vi "VI Gaszuordnung.vi"() -> ()   [LabVIEW 2020, in "Gaszuordnung AO.lvlib"]
uses:
  Seiten/Gaszuordnung AO/Gaszuordnung AO.lvlib
  Seiten/Gaszuordnung AO/Auswahlfelder Anzeige.ctl
  Visualisierungs Elemente/Auswahlfeld.ctl
  Seiten/Gaszuordnung AO/Aktuelle Werte Anzeige.ctl
  Seiten/Gaszuordnung AO/Grenzen Anzeige.ctl
  Visualisierungs Elemente/Zahlen-Eingabefeld.ctl
  Seiten/Gaszuordnung AO/Einheit Anzeige.ctl
  Visualisierungs Elemente/String - Ausgabefeld.ctl
  Seiten/Gaszuordnung AO/Balken Anzeige.ctl
  Seiten/Gaszuordnung AO/Balken.ctl
  Visualisierungs Elemente/Button.ctl
  Seiten/Gaszuordnung AO/FGV Gaszuordnung Gas-Auswahl Aktion.ctl
  Seiten/FT-IR/FGV FT-IR Gasliste Aktionen.ctl
  Passwortverwaltung/FGV Passwort Aktion.ctl
  Seiten/Gaszuordnung AO/FGV Gaszuordnung Grenzen&Einheit Aktion.ctl
  Seiten/FT-IR/FT-IR.lvlib
  Passwortverwaltung/Passwort.lvlib
  Allgemein/allgemeine Sub-VIs.lvlib
panel:
  in  "Grenzw. Speichern":T1
  in  "Grenzen Max":T2 {"Zahlen-Eingabefeld 16" format="%#_5g"; "Zahlen-Eingabefeld 15" format="%#_5g"; "Zahlen-Eingabefeld 14" format="%#_5g"; "Zahlen-Eingabefeld 13" format="%#_5g"; "Zahlen-Eingabefeld 12" format="%#_5g"; "Zahlen-Eingabefeld 11" format="%#_5g"; "Zahlen-Eingabefeld 10" format="%#_5g"; "Zahlen-Eingabefeld 9" format="%#_5g"; "Zahlen-Eingabefeld 8" format="%#_5g"; "Zahlen-Eingabefeld 7" format="%#_5g"; "Zahlen-Eingabefeld 6" format="%#_5g"; "Zahlen-Eingabefeld 5" format="%#_5g"; "Zahlen-Eingabefeld 4" format="%#_5g"; "Zahlen-Eingabefeld 3" format="%#_5g"; "Zahlen-Eingabefeld 2" format="%#_5g"; "Zahlen-Eingabefeld" format="%#_5g"}
  out "Balken Anzeige":T4 {"Anzeige Balken 16" scale=0.0..100.0; "Anzeige Balken 15" scale=0.0..100.0; "Anzeige Balken 14" scale=0.0..100.0; "Anzeige Balken 13" scale=0.0..100.0; "Anzeige Balken 12" scale=0.0..100.0; "Anzeige Balken 11" scale=0.0..100.0; "Anzeige Balken 10" scale=0.0..100.0; "Anzeige Balken 9" scale=0.0..100.0; "Anzeige Balken 8" scale=0.0..100.0; "Anzeige Balken 7" scale=0.0..100.0; "Anzeige Balken 6" scale=0.0..100.0; "Anzeige Balken 5" scale=0.0..100.0; "Anzeige Balken 4" scale=0.0..100.0; "Anzeige Balken 3" scale=0.0..100.0; "Anzeige Balken 2" scale=0.0..100.0; "Anzeige Balken" scale=0.0..100.0}
  out "Einheit Anzeige":T6
  in  "Grenzen Min":T2 {"Zahlen-Eingabefeld 16" format="%#_5g"; "Zahlen-Eingabefeld 15" format="%#_5g"; "Zahlen-Eingabefeld 14" format="%#_5g"; "Zahlen-Eingabefeld 13" format="%#_5g"; "Zahlen-Eingabefeld 12" format="%#_5g"; "Zahlen-Eingabefeld 11" format="%#_5g"; "Zahlen-Eingabefeld 10" format="%#_5g"; "Zahlen-Eingabefeld 9" format="%#_5g"; "Zahlen-Eingabefeld 8" format="%#_5g"; "Zahlen-Eingabefeld 7" format="%#_5g"; "Zahlen-Eingabefeld 6" format="%#_5g"; "Zahlen-Eingabefeld 5" format="%#_5g"; "Zahlen-Eingabefeld 4" format="%#_5g"; "Zahlen-Eingabefeld 3" format="%#_5g"; "Zahlen-Eingabefeld 2" format="%#_5g"; "Zahlen-Eingabefeld" format="%#_5g"}
  out "Aktuelle Werte":T8 {"Zahlen-Ausgabefeld 16" format="%#.2f"; "Zahlen-Ausgabefeld 15" format="%#.2f"; "Zahlen-Ausgabefeld 14" format="%#.2f"; "Zahlen-Ausgabefeld 13" format="%#.2f"; "Zahlen-Ausgabefeld 12" format="%#.2f"; "Zahlen-Ausgabefeld 11" format="%#.2f"; "Zahlen-Ausgabefeld 10" format="%#.2f"; "Zahlen-Ausgabefeld 9" format="%#.2f"; "Zahlen-Ausgabefeld 8" format="%#.2f"; "Zahlen-Ausgabefeld 7" format="%#.2f"; "Zahlen-Ausgabefeld 6" format="%#.2f"; "Zahlen-Ausgabefeld 5" format="%#.2f"; "Zahlen-Ausgabefeld 4" format="%#.2f"; "Zahlen-Ausgabefeld 3" format="%#.2f"; "Zahlen-Ausgabefeld 2" format="%#.2f"; "Zahlen-Ausgabefeld" format="%#.2f"}
  in  "Auswahlfelder":T9 {"Auswahl 16" items=["NO (3000) LP 191C", "NO2 (150) LP 191C (1of2)", "NO2 (2000) LP 191C (2of2)", "N2O (300) LP 191C (1of2)", "NH3 (300) LP 191C (1of2)", "NH3 (900,3000) LP 191C (2of2)", "HNCO (400) 191C", "H2O% (30) LP 191C", "Formaldehyde (70,500) LP 191C", "CO2 low% (4) LP 191C (2of2)", "CO2% (20) LP 191C (1of2)", "CO (700) LP 191C (1of3)", "CO% (1) LP 191C (2of3)", "Propylene (1000) LP 191C", "Aromatic HC C7 (500) LP 191C", "Ethylene (1000) LP 191C", "CH4 (250) LP 191C (1of2)", "CH4 (5000) LP 191C (2of2)", "Ethane (1000) LP 191C", "Acetylene (1000) LP 191C", "HNO2 (20) 191C", "MeOH (1000) 191C", "CO% (10) LP 191C (3of3)", "Formic Acid (100) 191C", "SO2 (500) LP 191C", "Acetaldehyde (1000) LP 191C", "COS (100) LP 191C", "1,3 butadiene (100) LP 191C", "Oil as Octane (200) LP 191C", "N2O (1000) LP 191C (2of2)", "Propane (200) LP 191C", "NO2 autorange (2000)", "CO autorange (100000)", "CH4 autorange (5000)", "NH3 autorange (3000)", "NOx autorange (3000)", "HCD (10000)", "NMHCD (10000)", "CO2% autorange (20)", "H2Oppm (300000)", "N2O autorange (1000)", "NMNEHCD (3000)", "Temp. Gascell", "Pressure Gascell", "sBeam@2500", "Temp. HL to FT-IR", "Temp. HL Extern SP1", "Outlet Temp FT-IR", "Temp. Cabinet", "Constant 0", "Constant 50", "Constant 100", "AK DUMMY"]; "Auswahl 15" items=["NO (3000) LP 191C", "NO2 (150) LP 191C (1of2)", "NO2 (2000) LP 191C (2of2)", "N2O (300) LP 191C (1of2)", "NH3 (300) LP 191C (1of2)", "NH3 (900,3000) LP 191C (2of2)", "HNCO (400) 191C", "H2O% (30) LP 191C", "Formaldehyde (70,500) LP 191C", "CO2 low% (4) LP 191C (2of2)", "CO2% (20) LP 191C (1of2)", "CO (700) LP 191C (1of3)", "CO% (1) LP 191C (2of3)", "Propylene (1000) LP 191C", "Aromatic HC C7 (500) LP 191C", "Ethylene (1000) LP 191C", "CH4 (250) LP 191C (1of2)", "CH4 (5000) LP 191C (2of2)", "Ethane (1000) LP 191C", "Acetylene (1000) LP 191C", "HNO2 (20) 191C", "MeOH (1000) 191C", "CO% (10) LP 191C (3of3)", "Formic Acid (100) 191C", "SO2 (500) LP 191C", "Acetaldehyde (1000) LP 191C", "COS (100) LP 191C", "1,3 butadiene (100) LP 191C", "Oil as Octane (200) LP 191C", "N2O (1000) LP 191C (2of2)", "Propane (200) LP 191C", "NO2 autorange (2000)", "CO autorange (100000)", "CH4 autorange (5000)", "NH3 autorange (3000)", "NOx autorange (3000)", "HCD (10000)", "NMHCD (10000)", "CO2% autorange (20)", "H2Oppm (300000)", "N2O autorange (1000)", "NMNEHCD (3000)", "Temp. Gascell", "Pressure Gascell", "sBeam@2500", "Temp. HL to FT-IR", "Temp. HL Extern SP1", "Outlet Temp FT-IR", "Temp. Cabinet", "Constant 0", "Constant 50", "Constant 100", "AK DUMMY"]; "Auswahl 14" items=["NO (3000) LP 191C", "NO2 (150) LP 191C (1of2)", "NO2 (2000) LP 191C (2of2)", "N2O (300) LP 191C (1of2)", "NH3 (300) LP 191C (1of2)", "NH3 (900,3000) LP 191C (2of2)", "HNCO (400) 191C", "H2O% (30) LP 191C", "Formaldehyde (70,500) LP 191C", "CO2 low% (4) LP 191C (2of2)", "CO2% (20) LP 191C (1of2)", "CO (700) LP 191C (1of3)", "CO% (1) LP 191C (2of3)", "Propylene (1000) LP 191C", "Aromatic HC C7 (500) LP 191C", "Ethylene (1000) LP 191C", "CH4 (250) LP 191C (1of2)", "CH4 (5000) LP 191C (2of2)", "Ethane (1000) LP 191C", "Acetylene (1000) LP 191C", "HNO2 (20) 191C", "MeOH (1000) 191C", "CO% (10) LP 191C (3of3)", "Formic Acid (100) 191C", "SO2 (500) LP 191C", "Acetaldehyde (1000) LP 191C", "COS (100) LP 191C", "1,3 butadiene (100) LP 191C", "Oil as Octane (200) LP 191C", "N2O (1000) LP 191C (2of2)", "Propane (200) LP 191C", "NO2 autorange (2000)", "CO autorange (100000)", "CH4 autorange (5000)", "NH3 autorange (3000)", "NOx autorange (3000)", "HCD (10000)", "NMHCD (10000)", "CO2% autorange (20)", "H2Oppm (300000)", "N2O autorange (1000)", "NMNEHCD (3000)", "Temp. Gascell", "Pressure Gascell", "sBeam@2500", "Temp. HL to FT-IR", "Temp. HL Extern SP1", "Outlet Temp FT-IR", "Temp. Cabinet", "Constant 0", "Constant 50", "Constant 100", "AK DUMMY"]; "Auswahl 13" items=["NO (3000) LP 191C", "NO2 (150) LP 191C (1of2)", "NO2 (2000) LP 191C (2of2)", "N2O (300) LP 191C (1of2)", "NH3 (300) LP 191C (1of2)", "NH3 (900,3000) LP 191C (2of2)", "HNCO (400) 191C", "H2O% (30) LP 191C", "Formaldehyde (70,500) LP 191C", "CO2 low% (4) LP 191C (2of2)", "CO2% (20) LP 191C (1of2)", "CO (700) LP 191C (1of3)", "CO% (1) LP 191C (2of3)", "Propylene (1000) LP 191C", "Aromatic HC C7 (500) LP 191C", "Ethylene (1000) LP 191C", "CH4 (250) LP 191C (1of2)", "CH4 (5000) LP 191C (2of2)", "Ethane (1000) LP 191C", "Acetylene (1000) LP 191C", "HNO2 (20) 191C", "MeOH (1000) 191C", "CO% (10) LP 191C (3of3)", "Formic Acid (100) 191C", "SO2 (500) LP 191C", "Acetaldehyde (1000) LP 191C", "COS (100) LP 191C", "1,3 butadiene (100) LP 191C", "Oil as Octane (200) LP 191C", "N2O (1000) LP 191C (2of2)", "Propane (200) LP 191C", "NO2 autorange (2000)", "CO autorange (100000)", "CH4 autorange (5000)", "NH3 autorange (3000)", "NOx autorange (3000)", "HCD (10000)", "NMHCD (10000)", "CO2% autorange (20)", "H2Oppm (300000)", "N2O autorange (1000)", "NMNEHCD (3000)", "Temp. Gascell", "Pressure Gascell", "sBeam@2500", "Temp. HL to FT-IR", "Temp. HL Extern SP1", "Outlet Temp FT-IR", "Temp. Cabinet", "Constant 0", "Constant 50", "Constant 100", "AK DUMMY"]; "Auswahl 12" items=["NO (3000) LP 191C", "NO2 (150) LP 191C (1of2)", "NO2 (2000) LP 191C (2of2)", "N2O (300) LP 191C (1of2)", "NH3 (300) LP 191C (1of2)", "NH3 (900,3000) LP 191C (2of2)", "HNCO (400) 191C", "H2O% (30) LP 191C", "Formaldehyde (70,500) LP 191C", "CO2 low% (4) LP 191C (2of2)", "CO2% (20) LP 191C (1of2)", "CO (700) LP 191C (1of3)", "CO% (1) LP 191C (2of3)", "Propylene (1000) LP 191C", "Aromatic HC C7 (500) LP 191C", "Ethylene (1000) LP 191C", "CH4 (250) LP 191C (1of2)", "CH4 (5000) LP 191C (2of2)", "Ethane (1000) LP 191C", "Acetylene (1000) LP 191C", "HNO2 (20) 191C", "MeOH (1000) 191C", "CO% (10) LP 191C (3of3)", "Formic Acid (100) 191C", "SO2 (500) LP 191C", "Acetaldehyde (1000) LP 191C", "COS (100) LP 191C", "1,3 butadiene (100) LP 191C", "Oil as Octane (200) LP 191C", "N2O (1000) LP 191C (2of2)", "Propane (200) LP 191C", "NO2 autorange (2000)", "CO autorange (100000)", "CH4 autorange (5000)", "NH3 autorange (3000)", "NOx autorange (3000)", "HCD (10000)", "NMHCD (10000)", "CO2% autorange (20)", "H2Oppm (300000)", "N2O autorange (1000)", "NMNEHCD (3000)", "Temp. Gascell", "Pressure Gascell", "sBeam@2500", "Temp. HL to FT-IR", "Temp. HL Extern SP1", "Outlet Temp FT-IR", "Temp. Cabinet", "Constant 0", "Constant 50", "Constant 100", "AK DUMMY"]; "Auswahl 11" items=["NO (3000) LP 191C", "NO2 (150) LP 191C (1of2)", "NO2 (2000) LP 191C (2of2)", "N2O (300) LP 191C (1of2)", "NH3 (300) LP 191C (1of2)", "NH3 (900,3000) LP 191C (2of2)", "HNCO (400) 191C", "H2O% (30) LP 191C", "Formaldehyde (70,500) LP 191C", "CO2 low% (4) LP 191C (2of2)", "CO2% (20) LP 191C (1of2)", "CO (700) LP 191C (1of3)", "CO% (1) LP 191C (2of3)", "Propylene (1000) LP 191C", "Aromatic HC C7 (500) LP 191C", "Ethylene (1000) LP 191C", "CH4 (250) LP 191C (1of2)", "CH4 (5000) LP 191C (2of2)", "Ethane (1000) LP 191C", "Acetylene (1000) LP 191C", "HNO2 (20) 191C", "MeOH (1000) 191C", "CO% (10) LP 191C (3of3)", "Formic Acid (100) 191C", "SO2 (500) LP 191C", "Acetaldehyde (1000) LP 191C", "COS (100) LP 191C", "1,3 butadiene (100) LP 191C", "Oil as Octane (200) LP 191C", "N2O (1000) LP 191C (2of2)", "Propane (200) LP 191C", "NO2 autorange (2000)", "CO autorange (100000)", "CH4 autorange (5000)", "NH3 autorange (3000)", "NOx autorange (3000)", "HCD (10000)", "NMHCD (10000)", "CO2% autorange (20)", "H2Oppm (300000)", "N2O autorange (1000)", "NMNEHCD (3000)", "Temp. Gascell", "Pressure Gascell", "sBeam@2500", "Temp. HL to FT-IR", "Temp. HL Extern SP1", "Outlet Temp FT-IR", "Temp. Cabinet", "Constant 0", "Constant 50", "Constant 100", "AK DUMMY"]; "Auswahl 10" items=["NO (3000) LP 191C", "NO2 (150) LP 191C (1of2)", "NO2 (2000) LP 191C (2of2)", "N2O (300) LP 191C (1of2)", "NH3 (300) LP 191C (1of2)", "NH3 (900,3000) LP 191C (2of2)", "HNCO (400) 191C", "H2O% (30) LP 191C", "Formaldehyde (70,500) LP 191C", "CO2 low% (4) LP 191C (2of2)", "CO2% (20) LP 191C (1of2)", "CO (700) LP 191C (1of3)", "CO% (1) LP 191C (2of3)", "Propylene (1000) LP 191C", "Aromatic HC C7 (500) LP 191C", "Ethylene (1000) LP 191C", "CH4 (250) LP 191C (1of2)", "CH4 (5000) LP 191C (2of2)", "Ethane (1000) LP 191C", "Acetylene (1000) LP 191C", "HNO2 (20) 191C", "MeOH (1000) 191C", "CO% (10) LP 191C (3of3)", "Formic Acid (100) 191C", "SO2 (500) LP 191C", "Acetaldehyde (1000) LP 191C", "COS (100) LP 191C", "1,3 butadiene (100) LP 191C", "Oil as Octane (200) LP 191C", "N2O (1000) LP 191C (2of2)", "Propane (200) LP 191C", "NO2 autorange (2000)", "CO autorange (100000)", "CH4 autorange (5000)", "NH3 autorange (3000)", "NOx autorange (3000)", "HCD (10000)", "NMHCD (10000)", "CO2% autorange (20)", "H2Oppm (300000)", "N2O autorange (1000)", "NMNEHCD (3000)", "Temp. Gascell", "Pressure Gascell", "sBeam@2500", "Temp. HL to FT-IR", "Temp. HL Extern SP1", "Outlet Temp FT-IR", "Temp. Cabinet", "Constant 0", "Constant 50", "Constant 100", "AK DUMMY"]; "Auswahl 9" items=["NO (3000) LP 191C", "NO2 (150) LP 191C (1of2)", "NO2 (2000) LP 191C (2of2)", "N2O (300) LP 191C (1of2)", "NH3 (300) LP 191C (1of2)", "NH3 (900,3000) LP 191C (2of2)", "HNCO (400) 191C", "H2O% (30) LP 191C", "Formaldehyde (70,500) LP 191C", "CO2 low% (4) LP 191C (2of2)", "CO2% (20) LP 191C (1of2)", "CO (700) LP 191C (1of3)", "CO% (1) LP 191C (2of3)", "Propylene (1000) LP 191C", "Aromatic HC C7 (500) LP 191C", "Ethylene (1000) LP 191C", "CH4 (250) LP 191C (1of2)", "CH4 (5000) LP 191C (2of2)", "Ethane (1000) LP 191C", "Acetylene (1000) LP 191C", "HNO2 (20) 191C", "MeOH (1000) 191C", "CO% (10) LP 191C (3of3)", "Formic Acid (100) 191C", "SO2 (500) LP 191C", "Acetaldehyde (1000) LP 191C", "COS (100) LP 191C", "1,3 butadiene (100) LP 191C", "Oil as Octane (200) LP 191C", "N2O (1000) LP 191C (2of2)", "Propane (200) LP 191C", "NO2 autorange (2000)", "CO autorange (100000)", "CH4 autorange (5000)", "NH3 autorange (3000)", "NOx autorange (3000)", "HCD (10000)", "NMHCD (10000)", "CO2% autorange (20)", "H2Oppm (300000)", "N2O autorange (1000)", "NMNEHCD (3000)", "Temp. Gascell", "Pressure Gascell", "sBeam@2500", "Temp. HL to FT-IR", "Temp. HL Extern SP1", "Outlet Temp FT-IR", "Temp. Cabinet", "Constant 0", "Constant 50", "Constant 100", "AK DUMMY"]; "Auswahl 8" items=["NO (3000) LP 191C", "NO2 (150) LP 191C (1of2)", "NO2 (2000) LP 191C (2of2)", "N2O (300) LP 191C (1of2)", "NH3 (300) LP 191C (1of2)", "NH3 (900,3000) LP 191C (2of2)", "HNCO (400) 191C", "H2O% (30) LP 191C", "Formaldehyde (70,500) LP 191C", "CO2 low% (4) LP 191C (2of2)", "CO2% (20) LP 191C (1of2)", "CO (700) LP 191C (1of3)", "CO% (1) LP 191C (2of3)", "Propylene (1000) LP 191C", "Aromatic HC C7 (500) LP 191C", "Ethylene (1000) LP 191C", "CH4 (250) LP 191C (1of2)", "CH4 (5000) LP 191C (2of2)", "Ethane (1000) LP 191C", "Acetylene (1000) LP 191C", "HNO2 (20) 191C", "MeOH (1000) 191C", "CO% (10) LP 191C (3of3)", "Formic Acid (100) 191C", "SO2 (500) LP 191C", "Acetaldehyde (1000) LP 191C", "COS (100) LP 191C", "1,3 butadiene (100) LP 191C", "Oil as Octane (200) LP 191C", "N2O (1000) LP 191C (2of2)", "Propane (200) LP 191C", "NO2 autorange (2000)", "CO autorange (100000)", "CH4 autorange (5000)", "NH3 autorange (3000)", "NOx autorange (3000)", "HCD (10000)", "NMHCD (10000)", "CO2% autorange (20)", "H2Oppm (300000)", "N2O autorange (1000)", "NMNEHCD (3000)", "Temp. Gascell", "Pressure Gascell", "sBeam@2500", "Temp. HL to FT-IR", "Temp. HL Extern SP1", "Outlet Temp FT-IR", "Temp. Cabinet", "Constant 0", "Constant 50", "Constant 100", "AK DUMMY"]; "Auswahl 7" items=["NO (3000) LP 191C", "NO2 (150) LP 191C (1of2)", "NO2 (2000) LP 191C (2of2)", "N2O (300) LP 191C (1of2)", "NH3 (300) LP 191C (1of2)", "NH3 (900,3000) LP 191C (2of2)", "HNCO (400) 191C", "H2O% (30) LP 191C", "Formaldehyde (70,500) LP 191C", "CO2 low% (4) LP 191C (2of2)", "CO2% (20) LP 191C (1of2)", "CO (700) LP 191C (1of3)", "CO% (1) LP 191C (2of3)", "Propylene (1000) LP 191C", "Aromatic HC C7 (500) LP 191C", "Ethylene (1000) LP 191C", "CH4 (250) LP 191C (1of2)", "CH4 (5000) LP 191C (2of2)", "Ethane (1000) LP 191C", "Acetylene (1000) LP 191C", "HNO2 (20) 191C", "MeOH (1000) 191C", "CO% (10) LP 191C (3of3)", "Formic Acid (100) 191C", "SO2 (500) LP 191C", "Acetaldehyde (1000) LP 191C", "COS (100) LP 191C", "1,3 butadiene (100) LP 191C", "Oil as Octane (200) LP 191C", "N2O (1000) LP 191C (2of2)", "Propane (200) LP 191C", "NO2 autorange (2000)", "CO autorange (100000)", "CH4 autorange (5000)", "NH3 autorange (3000)", "NOx autorange (3000)", "HCD (10000)", "NMHCD (10000)", "CO2% autorange (20)", "H2Oppm (300000)", "N2O autorange (1000)", "NMNEHCD (3000)", "Temp. Gascell", "Pressure Gascell", "sBeam@2500", "Temp. HL to FT-IR", "Temp. HL Extern SP1", "Outlet Temp FT-IR", "Temp. Cabinet", "Constant 0", "Constant 50", "Constant 100", "AK DUMMY"]; "Auswahl 6" items=["NO (3000) LP 191C", "NO2 (150) LP 191C (1of2)", "NO2 (2000) LP 191C (2of2)", "N2O (300) LP 191C (1of2)", "NH3 (300) LP 191C (1of2)", "NH3 (900,3000) LP 191C (2of2)", "HNCO (400) 191C", "H2O% (30) LP 191C", "Formaldehyde (70,500) LP 191C", "CO2 low% (4) LP 191C (2of2)", "CO2% (20) LP 191C (1of2)", "CO (700) LP 191C (1of3)", "CO% (1) LP 191C (2of3)", "Propylene (1000) LP 191C", "Aromatic HC C7 (500) LP 191C", "Ethylene (1000) LP 191C", "CH4 (250) LP 191C (1of2)", "CH4 (5000) LP 191C (2of2)", "Ethane (1000) LP 191C", "Acetylene (1000) LP 191C", "HNO2 (20) 191C", "MeOH (1000) 191C", "CO% (10) LP 191C (3of3)", "Formic Acid (100) 191C", "SO2 (500) LP 191C", "Acetaldehyde (1000) LP 191C", "COS (100) LP 191C", "1,3 butadiene (100) LP 191C", "Oil as Octane (200) LP 191C", "N2O (1000) LP 191C (2of2)", "Propane (200) LP 191C", "NO2 autorange (2000)", "CO autorange (100000)", "CH4 autorange (5000)", "NH3 autorange (3000)", "NOx autorange (3000)", "HCD (10000)", "NMHCD (10000)", "CO2% autorange (20)", "H2Oppm (300000)", "N2O autorange (1000)", "NMNEHCD (3000)", "Temp. Gascell", "Pressure Gascell", "sBeam@2500", "Temp. HL to FT-IR", "Temp. HL Extern SP1", "Outlet Temp FT-IR", "Temp. Cabinet", "Constant 0", "Constant 50", "Constant 100", "AK DUMMY"]; "Auswahl 5" items=["NO (3000) LP 191C", "NO2 (150) LP 191C (1of2)", "NO2 (2000) LP 191C (2of2)", "N2O (300) LP 191C (1of2)", "NH3 (300) LP 191C (1of2)", "NH3 (900,3000) LP 191C (2of2)", "HNCO (400) 191C", "H2O% (30) LP 191C", "Formaldehyde (70,500) LP 191C", "CO2 low% (4) LP 191C (2of2)", "CO2% (20) LP 191C (1of2)", "CO (700) LP 191C (1of3)", "CO% (1) LP 191C (2of3)", "Propylene (1000) LP 191C", "Aromatic HC C7 (500) LP 191C", "Ethylene (1000) LP 191C", "CH4 (250) LP 191C (1of2)", "CH4 (5000) LP 191C (2of2)", "Ethane (1000) LP 191C", "Acetylene (1000) LP 191C", "HNO2 (20) 191C", "MeOH (1000) 191C", "CO% (10) LP 191C (3of3)", "Formic Acid (100) 191C", "SO2 (500) LP 191C", "Acetaldehyde (1000) LP 191C", "COS (100) LP 191C", "1,3 butadiene (100) LP 191C", "Oil as Octane (200) LP 191C", "N2O (1000) LP 191C (2of2)", "Propane (200) LP 191C", "NO2 autorange (2000)", "CO autorange (100000)", "CH4 autorange (5000)", "NH3 autorange (3000)", "NOx autorange (3000)", "HCD (10000)", "NMHCD (10000)", "CO2% autorange (20)", "H2Oppm (300000)", "N2O autorange (1000)", "NMNEHCD (3000)", "Temp. Gascell", "Pressure Gascell", "sBeam@2500", "Temp. HL to FT-IR", "Temp. HL Extern SP1", "Outlet Temp FT-IR", "Temp. Cabinet", "Constant 0", "Constant 50", "Constant 100", "AK DUMMY"]; "Auswahl 4" items=["NO (3000) LP 191C", "NO2 (150) LP 191C (1of2)", "NO2 (2000) LP 191C (2of2)", "N2O (300) LP 191C (1of2)", "NH3 (300) LP 191C (1of2)", "NH3 (900,3000) LP 191C (2of2)", "HNCO (400) 191C", "H2O% (30) LP 191C", "Formaldehyde (70,500) LP 191C", "CO2 low% (4) LP 191C (2of2)", "CO2% (20) LP 191C (1of2)", "CO (700) LP 191C (1of3)", "CO% (1) LP 191C (2of3)", "Propylene (1000) LP 191C", "Aromatic HC C7 (500) LP 191C", "Ethylene (1000) LP 191C", "CH4 (250) LP 191C (1of2)", "CH4 (5000) LP 191C (2of2)", "Ethane (1000) LP 191C", "Acetylene (1000) LP 191C", "HNO2 (20) 191C", "MeOH (1000) 191C", "CO% (10) LP 191C (3of3)", "Formic Acid (100) 191C", "SO2 (500) LP 191C", "Acetaldehyde (1000) LP 191C", "COS (100) LP 191C", "1,3 butadiene (100) LP 191C", "Oil as Octane (200) LP 191C", "N2O (1000) LP 191C (2of2)", "Propane (200) LP 191C", "NO2 autorange (2000)", "CO autorange (100000)", "CH4 autorange (5000)", "NH3 autorange (3000)", "NOx autorange (3000)", "HCD (10000)", "NMHCD (10000)", "CO2% autorange (20)", "H2Oppm (300000)", "N2O autorange (1000)", "NMNEHCD (3000)", "Temp. Gascell", "Pressure Gascell", "sBeam@2500", "Temp. HL to FT-IR", "Temp. HL Extern SP1", "Outlet Temp FT-IR", "Temp. Cabinet", "Constant 0", "Constant 50", "Constant 100", "AK DUMMY"]; "Auswahl 3" items=["NO (3000) LP 191C", "NO2 (150) LP 191C (1of2)", "NO2 (2000) LP 191C (2of2)", "N2O (300) LP 191C (1of2)", "NH3 (300) LP 191C (1of2)", "NH3 (900,3000) LP 191C (2of2)", "HNCO (400) 191C", "H2O% (30) LP 191C", "Formaldehyde (70,500) LP 191C", "CO2 low% (4) LP 191C (2of2)", "CO2% (20) LP 191C (1of2)", "CO (700) LP 191C (1of3)", "CO% (1) LP 191C (2of3)", "Propylene (1000) LP 191C", "Aromatic HC C7 (500) LP 191C", "Ethylene (1000) LP 191C", "CH4 (250) LP 191C (1of2)", "CH4 (5000) LP 191C (2of2)", "Ethane (1000) LP 191C", "Acetylene (1000) LP 191C", "HNO2 (20) 191C", "MeOH (1000) 191C", "CO% (10) LP 191C (3of3)", "Formic Acid (100) 191C", "SO2 (500) LP 191C", "Acetaldehyde (1000) LP 191C", "COS (100) LP 191C", "1,3 butadiene (100) LP 191C", "Oil as Octane (200) LP 191C", "N2O (1000) LP 191C (2of2)", "Propane (200) LP 191C", "NO2 autorange (2000)", "CO autorange (100000)", "CH4 autorange (5000)", "NH3 autorange (3000)", "NOx autorange (3000)", "HCD (10000)", "NMHCD (10000)", "CO2% autorange (20)", "H2Oppm (300000)", "N2O autorange (1000)", "NMNEHCD (3000)", "Temp. Gascell", "Pressure Gascell", "sBeam@2500", "Temp. HL to FT-IR", "Temp. HL Extern SP1", "Outlet Temp FT-IR", "Temp. Cabinet", "Constant 0", "Constant 50", "Constant 100", "AK DUMMY"]; "Auswahl 2" items=["NO (3000) LP 191C", "NO2 (150) LP 191C (1of2)", "NO2 (2000) LP 191C (2of2)", "N2O (300) LP 191C (1of2)", "NH3 (300) LP 191C (1of2)", "NH3 (900,3000) LP 191C (2of2)", "HNCO (400) 191C", "H2O% (30) LP 191C", "Formaldehyde (70,500) LP 191C", "CO2 low% (4) LP 191C (2of2)", "CO2% (20) LP 191C (1of2)", "CO (700) LP 191C (1of3)", "CO% (1) LP 191C (2of3)", "Propylene (1000) LP 191C", "Aromatic HC C7 (500) LP 191C", "Ethylene (1000) LP 191C", "CH4 (250) LP 191C (1of2)", "CH4 (5000) LP 191C (2of2)", "Ethane (1000) LP 191C", "Acetylene (1000) LP 191C", "HNO2 (20) 191C", "MeOH (1000) 191C", "CO% (10) LP 191C (3of3)", "Formic Acid (100) 191C", "SO2 (500) LP 191C", "Acetaldehyde (1000) LP 191C", "COS (100) LP 191C", "1,3 butadiene (100) LP 191C", "Oil as Octane (200) LP 191C", "N2O (1000) LP 191C (2of2)", "Propane (200) LP 191C", "NO2 autorange (2000)", "CO autorange (100000)", "CH4 autorange (5000)", "NH3 autorange (3000)", "NOx autorange (3000)", "HCD (10000)", "NMHCD (10000)", "CO2% autorange (20)", "H2Oppm (300000)", "N2O autorange (1000)", "NMNEHCD (3000)", "Temp. Gascell", "Pressure Gascell", "sBeam@2500", "Temp. HL to FT-IR", "Temp. HL Extern SP1", "Outlet Temp FT-IR", "Temp. Cabinet", "Constant 0", "Constant 50", "Constant 100", "AK DUMMY"]; "Auswahl" items=["NO (3000) LP 191C", "NO2 (150) LP 191C (1of2)", "NO2 (2000) LP 191C (2of2)", "N2O (300) LP 191C (1of2)", "NH3 (300) LP 191C (1of2)", "NH3 (900,3000) LP 191C (2of2)", "HNCO (400) 191C", "H2O% (30) LP 191C", "Formaldehyde (70,500) LP 191C", "CO2 low% (4) LP 191C (2of2)", "CO2% (20) LP 191C (1of2)", "CO (700) LP 191C (1of3)", "CO% (1) LP 191C (2of3)", "Propylene (1000) LP 191C", "Aromatic HC C7 (500) LP 191C", "Ethylene (1000) LP 191C", "CH4 (250) LP 191C (1of2)", "CH4 (5000) LP 191C (2of2)", "Ethane (1000) LP 191C", "Acetylene (1000) LP 191C", "HNO2 (20) 191C", "MeOH (1000) 191C", "CO% (10) LP 191C (3of3)", "Formic Acid (100) 191C", "SO2 (500) LP 191C", "Acetaldehyde (1000) LP 191C", "COS (100) LP 191C", "1,3 butadiene (100) LP 191C", "Oil as Octane (200) LP 191C", "N2O (1000) LP 191C (2of2)", "Propane (200) LP 191C", "NO2 autorange (2000)", "CO autorange (100000)", "CH4 autorange (5000)", "NH3 autorange (3000)", "NOx autorange (3000)", "HCD (10000)", "NMHCD (10000)", "CO2% autorange (20)", "H2Oppm (300000)", "N2O autorange (1000)", "NMNEHCD (3000)", "Temp. Gascell", "Pressure Gascell", "sBeam@2500", "Temp. HL to FT-IR", "Temp. HL Extern SP1", "Outlet Temp FT-IR", "Temp. Cabinet", "Constant 0", "Constant 50", "Constant 100", "AK DUMMY"]}
  # "Gaszuordnung AO"
  # "Analogausgang\n(0-10V)"
  # "Komponente"
  # "Analogausgang in %"
  # "Aktueller Wert"
  # "MIN - MAX Wert"
  # "Einheit"
  # "Analogausgang 1:"
  # "Analogausgang 2:"
  # "Analogausgang 3:"
  # "Analogausgang 4:"
  # "Analogausgang 5:"
  # "Analogausgang 6:"
  # "Analogausgang 7:"
  # "Analogausgang 8:"
  # "Analogausgang 9:"
  # "Analogausgang 10:"
  # "Analogausgang 11:"
  # "Analogausgang 12:"
  # "Analogausgang 13:"
  # "Analogausgang 14:"
  # "Analogausgang 15:"
  # "Analogausgang 16:"
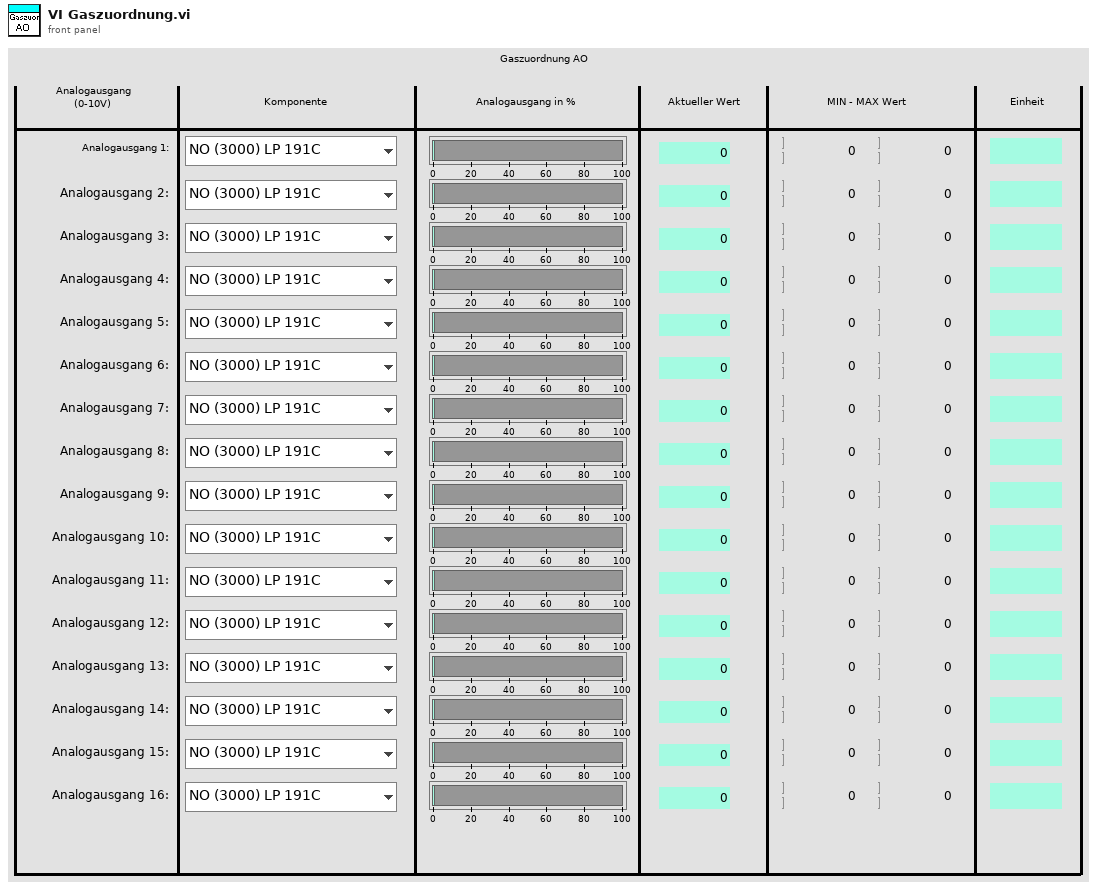
[diagram p1: front panel]
types:
  T1 = typedef "Button.ctl" = bool
  T2 = typedef "Gaszuordnung AO.lvlib/Grenzen Anzeige.ctl" = cluster{"Zahlen-Eingabefeld":T3, "Zahlen-Eingabefeld 2":T3, "Zahlen-Eingabefeld 3":T3, "Zahlen-Eingabefeld 4":T3, "Zahlen-Eingabefeld 5":T3, "Zahlen-Eingabefeld 6":T3, "Zahlen-Eingabefeld 7":T3, "Zahlen-Eingabefeld 8":T3, "Zahlen-Eingabefeld 9":T3, "Zahlen-Eingabefeld 10":T3, "Zahlen-Eingabefeld 11":T3, "Zahlen-Eingabefeld 12":T3, "Zahlen-Eingabefeld 13":T3, "Zahlen-Eingabefeld 14":T3, "Zahlen-Eingabefeld 15":T3, "Zahlen-Eingabefeld 16":T3}
  T3 = typedef "Zahlen-Eingabefeld.ctl" = sgl
  T4 = typedef "Gaszuordnung AO.lvlib/Balken Anzeige.ctl" = cluster{"Anzeige Balken":T5, "Anzeige Balken 2":T5, "Anzeige Balken 3":T5, "Anzeige Balken 4":T5, "Anzeige Balken 5":T5, "Anzeige Balken 6":T5, "Anzeige Balken 7":T5, "Anzeige Balken 8":T5, "Anzeige Balken 9":T5, "Anzeige Balken 10":T5, "Anzeige Balken 11":T5, "Anzeige Balken 12":T5, "Anzeige Balken 13":T5, "Anzeige Balken 14":T5, "Anzeige Balken 15":T5, "Anzeige Balken 16":T5}
  T5 = typedef "Gaszuordnung AO.lvlib/Balken.ctl" = u8
  T6 = typedef "Gaszuordnung AO.lvlib/Einheit Anzeige.ctl" = cluster{"String - Ausgabefeld":T7, "String - Ausgabefeld 2":T7, "String - Ausgabefeld 3":T7, "String - Ausgabefeld 4":T7, "String - Ausgabefeld 5":T7, "String - Ausgabefeld 6":T7, "String - Ausgabefeld 7":T7, "String - Ausgabefeld 8":T7, "String - Ausgabefeld 9":T7, "String - Ausgabefeld 10":T7, "String - Ausgabefeld 11":T7, "String - Ausgabefeld 12":T7, "String - Ausgabefeld 13":T7, "String - Ausgabefeld 14":T7, "String - Ausgabefeld 15":T7, "String - Ausgabefeld 16":T7}
  T7 = typedef "String - Ausgabefeld.ctl" = string
  T8 = typedef "Gaszuordnung AO.lvlib/Aktuelle Werte Anzeige.ctl" = cluster{"Zahlen-Ausgabefeld":sgl, "Zahlen-Ausgabefeld 2":sgl, "Zahlen-Ausgabefeld 3":sgl, "Zahlen-Ausgabefeld 4":sgl, "Zahlen-Ausgabefeld 5":sgl, "Zahlen-Ausgabefeld 6":sgl, "Zahlen-Ausgabefeld 7":sgl, "Zahlen-Ausgabefeld 8":sgl, "Zahlen-Ausgabefeld 9":sgl, "Zahlen-Ausgabefeld 10":sgl, "Zahlen-Ausgabefeld 11":sgl, "Zahlen-Ausgabefeld 12":sgl, "Zahlen-Ausgabefeld 13":sgl, "Zahlen-Ausgabefeld 14":sgl, "Zahlen-Ausgabefeld 15":sgl, "Zahlen-Ausgabefeld 16":sgl}
  T9 = typedef "Gaszuordnung AO.lvlib/Auswahlfelder Anzeige.ctl" = cluster{"Auswahl":T10, "Auswahl 2":T10, "Auswahl 3":T10, "Auswahl 4":T10, "Auswahl 5":T10, "Auswahl 6":T10, "Auswahl 7":T10, "Auswahl 8":T10, "Auswahl 9":T10, "Auswahl 10":T10, "Auswahl 11":T10, "Auswahl 12":T10, "Auswahl 13":T10, "Auswahl 14":T10, "Auswahl 15":T10, "Auswahl 16":T10}
  T10 = typedef "Auswahlfeld.ctl" = u16
  T11 = typedef "Gaszuordnung AO.lvlib/FGV Gaszuordnung Gas-Auswahl Aktion.ctl" = enum16{"Lesen", "AO Auswahl", "Graph Auswahl", "aktiver Graph", "laden", "speichern"}
  T12 = typedef "FT-IR.lvlib/FGV FT-IR Gasliste Aktionen.ctl" = enum16{"lesen", "Gasliste FT-IR", "Gasliste ausgelesen", "laden", "speichern", "löschen"}
  T13 = typedef "Passwort.lvlib/FGV Passwort Aktion.ctl" = enum16{"prüfen", "setzen", "Initialisieren", "PW speichern", "lesen", "PW Änderung"}
  T14 = typedef "Gaszuordnung AO.lvlib/FGV Gaszuordnung Grenzen&Einheit Aktion.ctl" = enum16{"Lesen", "Schreiben Min", "Schreiben Max", "Laden", "Speichern"}
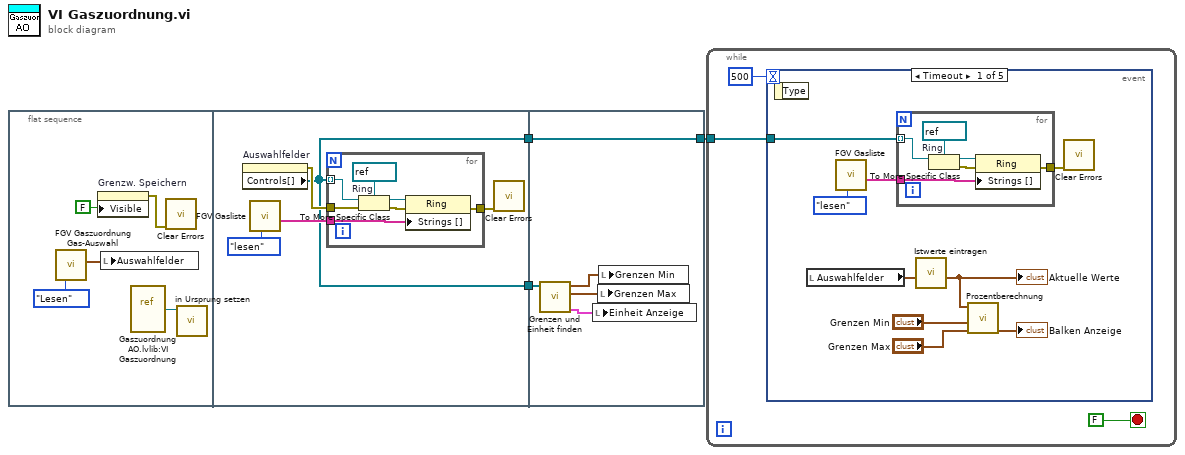
[diagram p0: block diagram]
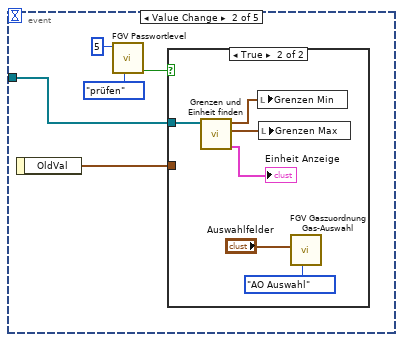
[diagram p2: hidden frame]
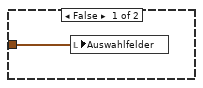
[diagram p3: hidden frame]
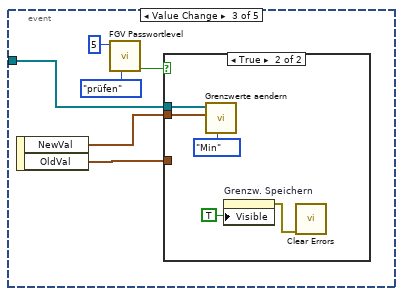
[diagram p4: hidden frame]
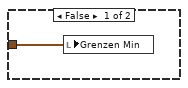
[diagram p5: hidden frame]
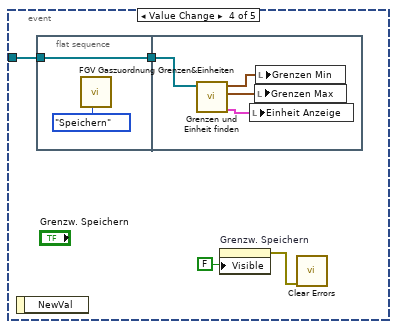
[diagram p6: hidden frame]
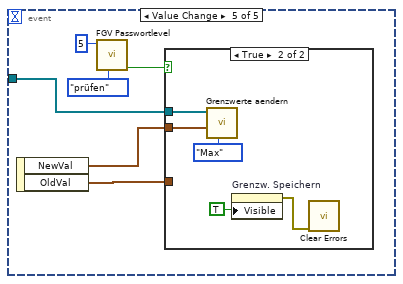
[diagram p7: hidden frame]
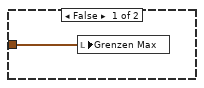
[diagram p8: hidden frame]
diagram:
  n1 = flat-sequence {
    tunnel: [w9] -> w2
    tunnel: [w9] -> w1
    tunnel: [w25] -> w3
    tunnel: w2 -> [w25]
    tunnel: w1 -> [w21]
    frame #0 {
      n2 = call "FGV Gaszuordnung Gas-Auswahl.vi"("Aktion"=FGV_Gaszuordnung_Gas-Auswahl_Aktion."Lesen") -> ("Auswahlfelder OUT"=w8:T9)  [unwired: 3 in, 7 out]
      n3 = property on="Grenzw. Speichern" class="Bool."("Visible"=FALSE ("Sichtbar")) -> (error out=w6:errorcluster)  [unwired: 2 in, 1 out]
      n4 = local write "Auswahlfelder"(w8) -> ()
      n5 = vi-ref "Gaszuordnung AO.lvlib:VI Gaszuordnung.vi"() -> (w4:refnum<vi>)
      n6 = call <vilib>:"Clear Errors.vi"("error in (no error)"=w6) -> ()  [unwired: 5 in, 2 out]
      n7 = call "in Ursprung setzen.vi"("VI Referenz"=w4) -> ()  [unwired: 10 in, 1 out]
    }
    frame #1 {
      n8 = property on="Auswahlfelder" class="Cluster (strikt)"() -> (error out=w13:errorcluster, "Controls[]"=w9:refnum<vi>[])  [unwired: 2 in, 1 out]
      n9 = call "FGV Gasliste.vi"("Aktionen"=FGV_FT-IR_Gasliste_Aktionen."lesen") -> ("Aktuelle Gasliste gesamt"=w11:T7[])  [unwired: 8 in, 2 out]
      n10 = for {
        tunnel: w9 -> [w19] mode=indexing
        tunnel: w11 -> [w17]
        tunnel: w13 -> [w16]
        tunnel: [w14] -> w10
        w20 = refnum<vi> refnum  # Ring
        n11 = To More Specific Class(target class=w20, reference=w19, error in=w16) -> (specific class reference=w18:refnum<vi>, error out=w15:errorcluster)
        n12 = property class="Ring"(reference=w18, error in=w15, "Strings []"=w17) -> (error out=w14:errorcluster)  [unwired: 1 out]
      }
      n13 = call <vilib>:"Clear Errors.vi"("error in (no error)"=w10) -> ()  [unwired: 5 in, 2 out]
    }
    frame #2 {
      n14 = call "Grenzen und Einheit finden.vi"("Ref Auswahlfelder"=w21) -> ("Einheit Anzeige"=w22:T6, "Grenzen Max"=w23:T2, "Grenzen Min"=w24:T2)  [unwired: 8 out]
      n15 = local write "Einheit Anzeige"(w22) -> ()
      n16 = local write "Grenzen Max"(w23) -> ()
      n17 = local write "Grenzen Min"(w24) -> ()
    }
  }
  n18 = while {
    tunnel: w3 -> [w26]
    stop <- FALSE stop-if-true
    n19 = event shown="[0] Timeout" {
      selector: _ -> [_ _ _ _ _]
      dyn-events: _ -> [_ _ _ _ _]
      timeout: 500 -> [_ _ _ _ _]
      tunnel: w26 -> [w34 w44 w56 w69 w78]
      event Timeout {
        n20 = event-data() -> ()  [unwired: 2 out]
        n21 = local read "Auswahlfelder"() -> (w29:T9)
        n22 = call "FGV Gasliste.vi"("Aktionen"=FGV_FT-IR_Gasliste_Aktionen."lesen") -> ("Aktuelle Gasliste gesamt"=w36:T7[])  [unwired: 8 in, 2 out]
        n23 = for {
          tunnel: w34 -> [w42] mode=indexing
          tunnel: w36 -> [w40]
          tunnel: [w38] -> w37
          w43 = refnum<vi> refnum  # Ring
          n24 = To More Specific Class(target class=w43, reference=w42) -> (specific class reference=w41:refnum<vi>, error out=w39:errorcluster)  [unwired: 1 in]
          n25 = property class="Ring"(reference=w41, error in=w39, "Strings []"=w40) -> (error out=w38:errorcluster)  [unwired: 1 out]
        }
        n26 = call "Istwerte eintragen.vi"("Auswahlfelder"=w29) -> ("Aktuelle Werte"=w32:T8)  [unwired: 2 in, 8 out]
        "Aktuelle Werte" <- w32
        n27 = call "Prozentberechnung.vi"("Grenzen Max"="Grenzen Max", "Grenzen Min"="Grenzen Min", "Aktuelle Werte"=w32) -> ("Balken Anzeige"=→"Balken Anzeige":T4)  [unwired: 1 in, 7 out]
        n28 = call <vilib>:"Clear Errors.vi"("error in (no error)"=w37) -> ()  [unwired: 5 in, 2 out]
      }
      event Value Change {
        n29 = event-data() -> ("OldVal"=w45:T9)  [unwired: 1 out]
        n30 = call "FGV Passwortlevel.vi"("FGV Passwort Aktion"=FGV_Passwort_Aktion."prüfen", "geforderter Level"=i16 5) -> ("Freigabe"=w46:bool)  [unwired: 2 in, 7 out]
        n31 = case shown="True" w46 {
          tunnel: w44 -> [_ w52]
          tunnel: w45 -> [w49 _]
          frame False {
            n32 = local write "Auswahlfelder"(w49) -> ()
          }
          frame True {
            n33 = call "Grenzen und Einheit finden.vi"("Ref Auswahlfelder"=w52) -> ("Einheit Anzeige"=→"Einheit Anzeige":T6, "Grenzen Max"=w53:T2, "Grenzen Min"=w54:T2)  [unwired: 8 out]
            n34 = local write "Grenzen Min"(w54) -> ()
            n35 = local write "Grenzen Max"(w53) -> ()
            n36 = call "FGV Gaszuordnung Gas-Auswahl.vi"("Aktion"=FGV_Gaszuordnung_Gas-Auswahl_Aktion."AO Auswahl", "Auswahlfelder"="Auswahlfelder") -> ()  [unwired: 2 in, 8 out]
          }
        }
      }
      event Value Change {
        n37 = event-data() -> ("NewVal"=w61:T2, "OldVal"=w57:T2)  [unwired: 1 out]
        n38 = call "FGV Passwortlevel.vi"("FGV Passwort Aktion"=FGV_Passwort_Aktion."prüfen", "geforderter Level"=i16 5) -> ("Freigabe"=w58:bool)  [unwired: 2 in, 7 out]
        n39 = case shown="True" w58 {
          tunnel: w61 -> [_ w67]
          tunnel: w56 -> [_ w65]
          tunnel: w57 -> [w62 _]
          frame False {
            n40 = local write "Grenzen Min"(w62) -> ()
          }
          frame True {
            n41 = call "Grenzwerte aendern.vi"("Auswahl"=enum16{"Min", "Max"}."Min", "Grenzen Min"=w67, "Ref Auswahlfelder"=w65) -> ()  [unwired: 1 in, 8 out]
            n42 = property on="Grenzw. Speichern" class="Bool."("Visible"=TRUE ("Sichtbar")) -> (error out=w63:errorcluster)  [unwired: 2 in, 1 out]
            n43 = call <vilib>:"Clear Errors.vi"("error in (no error)"=w63) -> ()  [unwired: 5 in, 2 out]
          }
        }
      }
      event Value Change {
        n44 = event-data() -> ()  [unwired: 2 out]
        n45 = flat-sequence {
          tunnel: [w72] -> w70
          tunnel: w69 -> [w72]
          tunnel: w70 -> [w74]
          frame #0 {
            n46 = call "FGV Gaszuordnung Grenzen&Einheiten.vi"("Aktion"=FGV_Gaszuordnung_Grenzen&Einheit_Aktion."Speichern") -> ()  [unwired: 7 in, 4 out]
          }
          frame #1 {
            n47 = call "Grenzen und Einheit finden.vi"("Ref Auswahlfelder"=w74) -> ("Einheit Anzeige"=w75:T6, "Grenzen Max"=w76:T2, "Grenzen Min"=w77:T2)  [unwired: 8 out]
            n48 = local write "Einheit Anzeige"(w75) -> ()
            n49 = local write "Grenzen Max"(w76) -> ()
            n50 = local write "Grenzen Min"(w77) -> ()
          }
        }
        n51 = property on="Grenzw. Speichern" class="Bool."("Visible"=FALSE ("Sichtbar")) -> (error out=w68:errorcluster)  [unwired: 2 in, 1 out]
        n52 = call <vilib>:"Clear Errors.vi"("error in (no error)"=w68) -> ()  [unwired: 5 in, 2 out]
      }
      event Value Change {
        n53 = event-data() -> ("NewVal"=w79:T2, "OldVal"=w80:T2)  [unwired: 1 out]
        n54 = call "FGV Passwortlevel.vi"("FGV Passwort Aktion"=FGV_Passwort_Aktion."prüfen", "geforderter Level"=i16 5) -> ("Freigabe"=w81:bool)  [unwired: 2 in, 7 out]
        n55 = case shown="True" w81 {
          tunnel: w78 -> [_ w88]
          tunnel: w80 -> [w84 _]
          tunnel: w79 -> [_ w86]
          frame False {
            n56 = local write "Grenzen Max"(w84) -> ()
          }
          frame True {
            n57 = call "Grenzwerte aendern.vi"("Auswahl"=enum16{"Min", "Max"}."Max", "Grenzen Max"=w86, "Ref Auswahlfelder"=w88) -> ()  [unwired: 1 in, 8 out]
            n58 = property on="Grenzw. Speichern" class="Bool."("Visible"=TRUE ("Sichtbar")) -> (error out=w85:errorcluster)  [unwired: 2 in, 1 out]
            n59 = call <vilib>:"Clear Errors.vi"("error in (no error)"=w85) -> ()  [unwired: 5 in, 2 out]
          }
        }
      }
    }
  }
